vi "Mecanum_drive_edit.vi"(5 "practice bot":bool=TRUE, 6 "Rotation":dbl, 7 "Gyro Angle":dbl, 8 "error in (no error)":errorcluster, 9 "Y":dbl, 10 "X":dbl, 11 "RobotDriveDevRef":T1={"DevStatus"={"status"=FALSE, "code"=0, "source"=""}, "Motors[]"=[], "Square Inputs"=FALSE, "Max Output"=1.0}) -> (0 "error out":errorcluster, 2 "Motor Values":dbl[](array[numeric]), 3 "RobotDriveDevRef":T1={"DevStatus"={"status"=FALSE, "code"=0, "source"=""}, "Motors[]"=[], "Square Inputs"=FALSE, "Max Output"=1.0})   [LabVIEW 2014]
doc: "Configures the motors for holonomic driving. Holonomic driving allows you to move the robot in any direction without first rotating or maneuvering the robot.\n\nThis VI requires the robot to have either four omni-directional wheels and four motors mounted at 45 degree angles in the four corners of a square frame or to have four mecanum wheels driven by four motors.\n\nThe control input is intended to be connected directly to the X, Y, and Z axes of a joystick. The Y axis is inverted for you.\n\nThis software is licensed. Open the labview\\readme\\WPI Robotics Library Open Source License.txt file for more information."
uses:
  <vilib>/Rock Robotics/WPI/RobotDrive/WPI_RobotDriveDevRef.ctl
  <vilib>/Rock Robotics/WPI/MotorControl/WPI_MotorControlDeviceRef.ctl
  <vilib>/Rock Robotics/WPI/MotorControl/WPI_MotorControlType.ctl
  <vilib>/Rock Robotics/SystemInterfaces/Typedef/FPGA_TypedefDigitalModule.ctl
  <vilib>/Rock Robotics/SystemInterfaces/DIO/FPGA_DIOPWMChannel.ctl
  <vilib>/Rock Robotics/WPI/PWM/WPI_PWMDeadband.ctl
  <vilib>/Rock Robotics/WPI/CAN/Jaguar/SubVIs/WPI_CANJaguar_ControlMode.ctl
  <vilib>/Rock Robotics/WPI/CAN/TalonSRX/WPI_CANTalonSRX_APIControlMode.ctl
  <vilib>/Rock Robotics/WPI/PWM/WPI_PWMTransform_ConPane.ctl
  <vilib>/Rock Robotics/SystemInterfaces/NetworkCommunication/NetComm_UsageReport_ResourceType.ctl
  <vilib>/Rock Robotics/WPI/RobotDrive/WPI_RobotDriveMotorSelectorEnum.ctl
  <vilib>/Rock Robotics/WPI/Joystick/WPI_JoystickGetSetRefNum.vi
  <vilib>/Rock Robotics/WPI/RobotDrive/WPI_RobotDriveSafetyCheck.vi
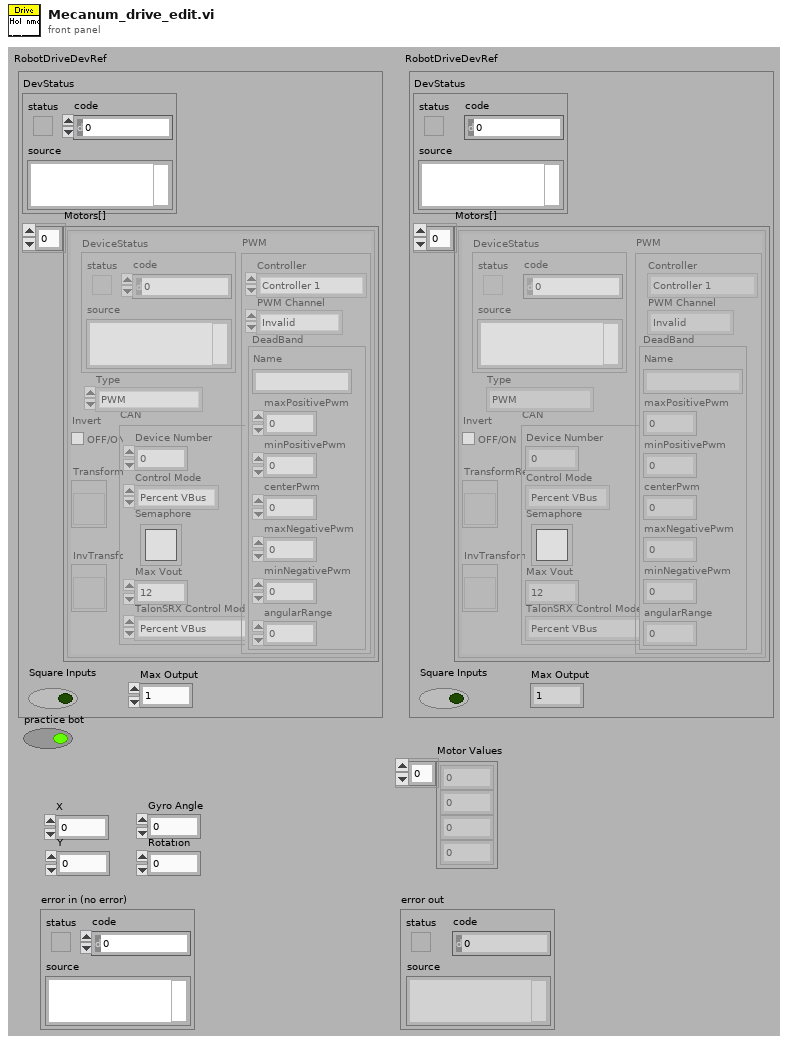
[diagram p1: front panel]
types:
  T1 = typedef "WPI_RobotDriveDevRef.ctl" = cluster{"DevStatus":errorcluster, "Motors[]":T2[], "Square Inputs":bool, "Max Output":dbl}
  T2 = typedef "WPI_MotorControlDeviceRef.ctl" = cluster{"DeviceStatus":errorcluster, "Type":T3, "PWM":cluster{"Controller":T4, "PWM Channel":T5, "DeadBand":T6}, "CAN":cluster{"Device Number":u8, "Control Mode":T7, "Semaphore":T8, "Max Vout":dbl, "TalonSRX Control Mode":T9}, "Invert":bool, "TransformRef":T10, "InvTransformRef":T10}
  T3 = typedef "WPI_MotorControlType.ctl" = enum16{"PWM", "CAN", "CANTalonSRX"}
  T4 = typedef "FPGA_TypedefDigitalModule.ctl" = enum16{"Controller 1"}
  T5 = typedef "FPGA_DIOPWMChannel.ctl" = enum8{"PWM 0", "PWM 1", "PWM 2", "PWM 3", "PWM 4", "PWM 5", "PWM 6", "PWM 7", "PWM 8", "PWM 9", "PWM MXP 0", "PWM MXP 1", "PWM MXP 2", "PWM MXP 3", "PWM MXP 4", "PWM MXP 5", "PWM MXP 6", "PWM MXP 7", "PWM MXP 8", "PWM MXP 9", "Invalid"}
  T6 = typedef "WPI_PWMDeadband.ctl" = cluster{"Name":string, "maxPositivePwm":i32, "minPositivePwm":i32, "centerPwm":i32, "maxNegativePwm":i32, "minNegativePwm":i32, "angularRange":u16}
  T7 = typedef "WPI_CANJaguar_ControlMode.ctl" = enum8{"Percent VBus", "Current", "Speed", "Position", "Voltage"}
  T8 = typedef "Semaphore RefNum" = refnum<k1>
  T9 = typedef "WPI_CANTalonSRX_APIControlMode.ctl" = enum8{"Percent VBus", "Speed", "Position", "Slave", "Unchanged / Invalid"}
  T10 = typedef "WPI_PWMTransform_ConPane.ctl" = refnum<vi>
  T11 = typedef "NetComm_UsageReport_ResourceType.ctl" = enum8{"Controller", "Module", "Language", "CANPlugin", "Accelerometer", "ADXL345", "AnalogChannel", "AnalogTrigger", "AnalogTriggerOutput", "CANJaguar", "Compressor", "Counter", "Dashboard", "DigitalInput", "DigitalOutput", "DriverStationCIO", "DriverStationEIO", "DriverStationLCD", "Encoder", "GearTooth", "Gyro", "I2C", "Framework", "Jaguar", "Joystick", "Kinect", "KinectStick", "PIDController", "Preferences", "PWM", "Relay", "RobotDrive", "SerialPort", "Servo", "Solenoid", "SPI", "Task", "Ultrasonic", "Victor", "Button", "Command", "AxisCamera", "PCVideoServer", "SmartDashboard", "Talon", "HiTechnicColorSensor", "HiTechnicAccel", "HiTechnicCompass", "SRF08", "AnalogOutput", "Victor SP", "Talon SRX", "CAN Talon SRX"}
  T12 = typedef "WPI_RobotDriveMotorSelectorEnum.ctl" = enum16{"Rear Left Motor", "Rear Right Motor", "Front Left Motor", "Front Right Motor"}
  T13 = typedef "WPI_JoystickDevRef.ctl" = cluster{"Device":T14}
  T14 = typedef "WPI_JoystickDeviceEnum.ctl" = enum16{"USB 0", "USB 1", "USB 2", "USB 3", "USB 4", "USB 5"}
  T15 = cluster{"Axes[0]":dbl, "Axes[1]":dbl, "Axes[2]":dbl, "Axes[3]":dbl, "Axes[4]":dbl, "Axes[5]":dbl, "Axes[6]":dbl, "Axes[7]":dbl, "Axes[8]":dbl}
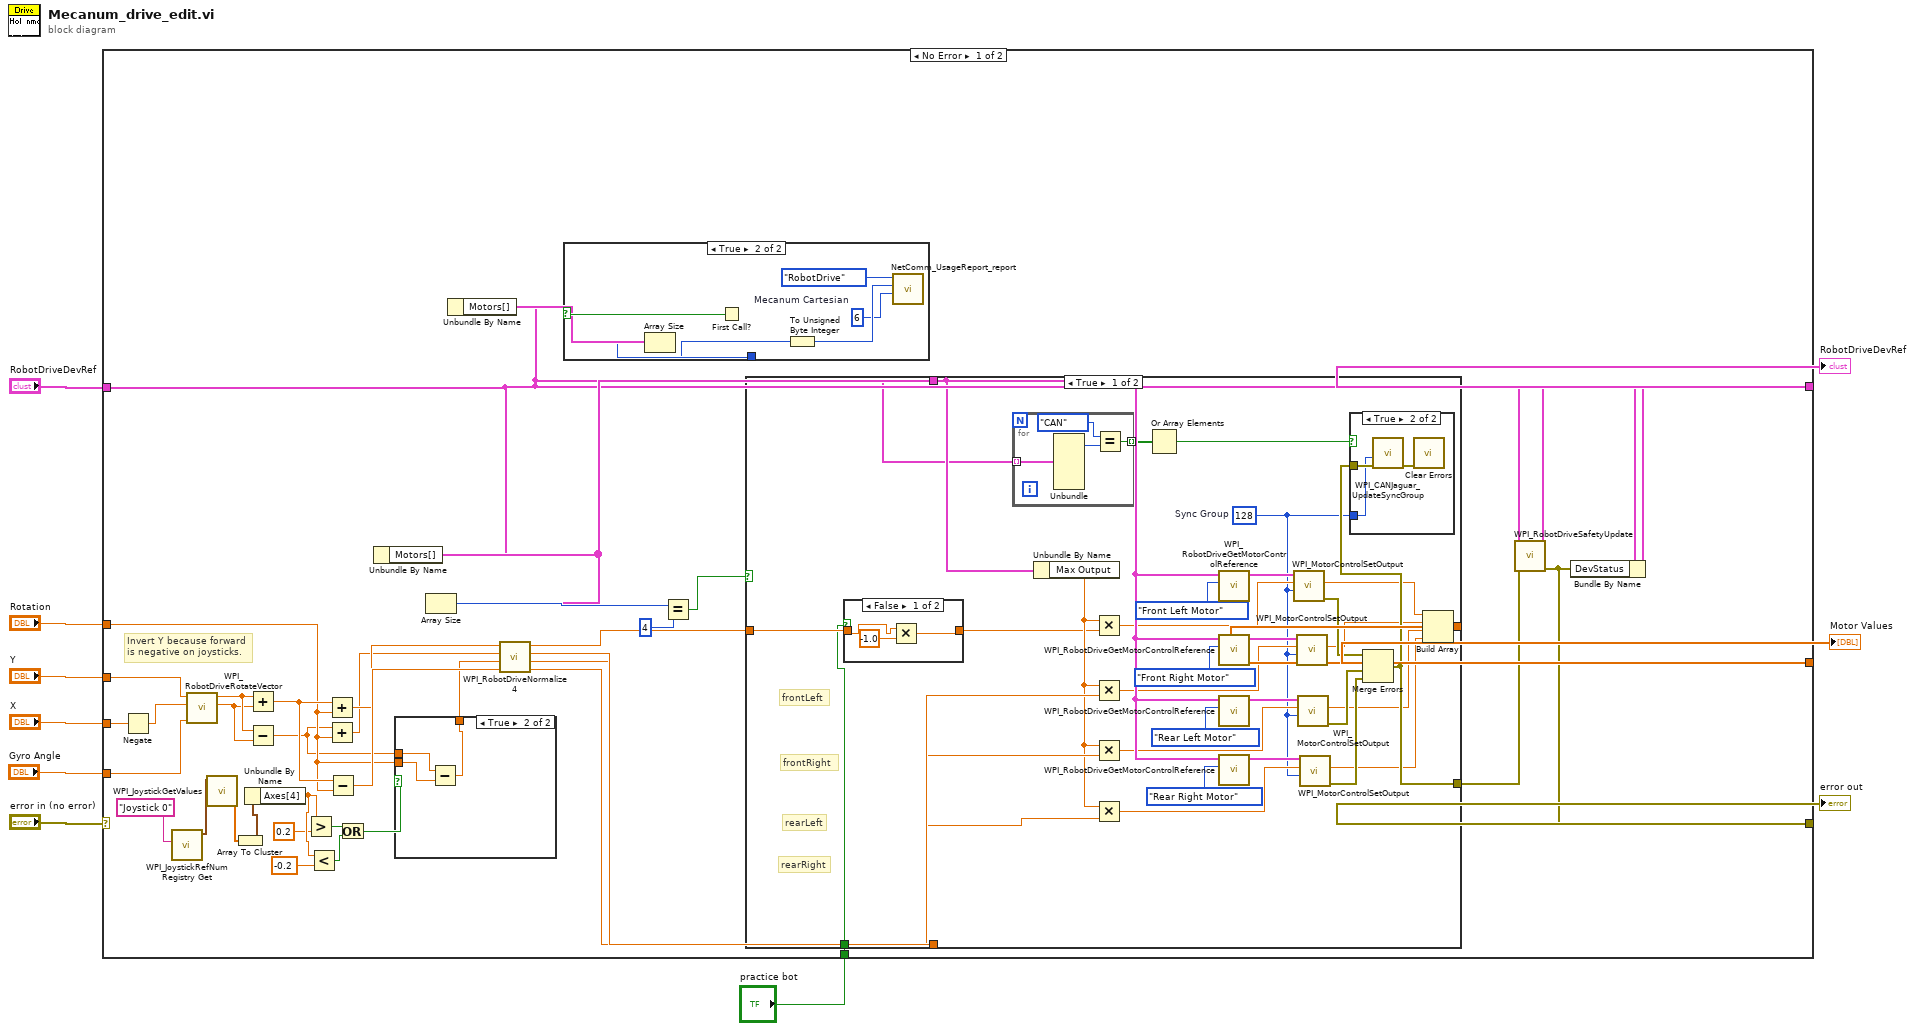
[diagram p0: block diagram]
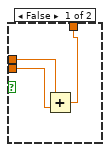
[diagram p2: hidden frame]
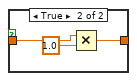
[diagram p4: hidden frame]
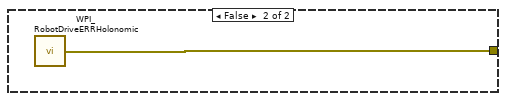
[diagram p6: hidden frame]
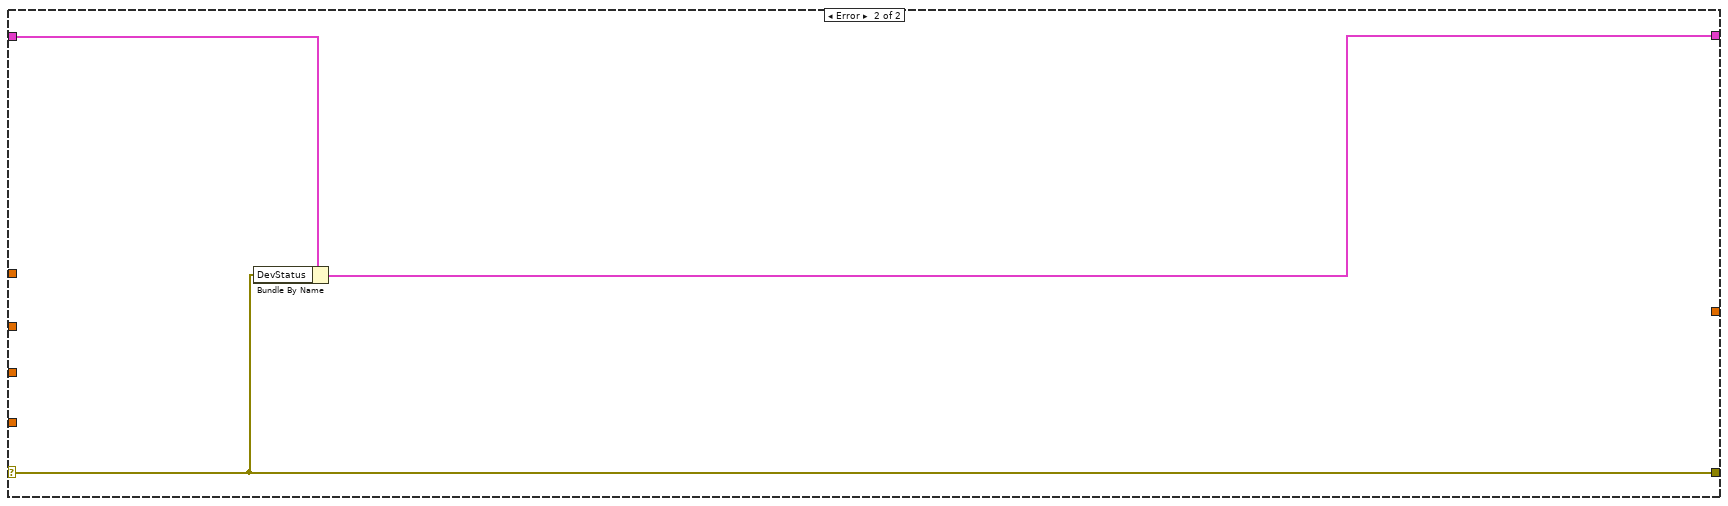
[diagram p7: hidden frame]
diagram:
  n1 = case shown="No Error" "error in (no error)" {
    selector: "error in (no error)" -> [_ w110]
    tunnel: "Y" -> [w14 _]
    tunnel: "X" -> [w12 _]
    tunnel: "RobotDriveDevRef" -> [w32 w112]
    tunnel: [w48 w111] -> w6
    tunnel: [w37 w110] -> w5
    tunnel: "Rotation" -> [w16 _]
    tunnel: "Gyro Angle" -> [w27 _]
    tunnel: [w31 _] -> w2
    tunnel: "practice bot" -> [w11 _]
    frame No Error {
      # "Invert Y because forward is negative on joysticks."
      n2 = Negate(x=w12) -> (-x=w13:dbl)
      n3 = call <vilib>:"WPI_JoystickRefNum Registry Get.vi"("refnum name"="Joystick 0") -> ("JoystickDevRef"=w29:T13)  [unwired: 9 in, 1 out]
      n4 = call <vilib>:"WPI_RobotDriveRotateVector.vi"("Angle"=w27, "X"=w13, "Y"=w14) -> ("X'"=w46:dbl, "Y'"=w47:dbl)  [unwired: 7 out]
      n5 = call <vilib>:"WPI_JoystickGetValues.vi"("JoystickDevRef"=w29) -> ("Axes"=w24:dbl[])  [unwired: 6 in, 4 out]
      n6 = Array To Cluster(array=w24) -> (cluster=w23:T15)
      n7 = Unbundle By Name(w23) -> ("Axes[4]"=w22:dbl)
      n8 = Add(x=w47, y=w46) -> (x+y=w19:dbl)
      n9 = Subtract(x=w47, y=w46) -> (x-y=w15:dbl)
      n10 = Greater?(x=w22, y=0.2) -> (0:w26:bool)
      n11 = Less?(x=w22, y=-0.2) -> (x < y?=w25:bool)
      n12 = Add(x=w19, y=w16) -> (x+y=w44:dbl)
      n13 = Add(x=w15, y=w16) -> (x+y=w30:dbl)
      n14 = Subtract(x=w19, y=w16) -> (x-y=w45:dbl)
      n15 = Or(x=w26, y=w25) -> (x .or. y?=w18:bool)
      n16 = Unbundle By Name(w32) -> ("Motors[]"=w36:T2[])
      n17 = case shown="True" w18 {
        tunnel: [w54 w55] -> w17
        tunnel: w16 -> [w53 w56]
        tunnel: w15 -> [w52 w57]
        frame False {
          n18 = Add(x=w52, y=w53) -> (x+y=w54:dbl)
        }
        frame True {
          n19 = Subtract(x=w57, y=w56) -> (x-y=w55:dbl)
        }
      }
      n20 = Array Size(array=w36) -> (size(s)=w51:i32)
      n21 = Unbundle By Name(w32) -> ("Motors[]"=w34:T2[])
      n22 = call <vilib>:"WPI_RobotDriveNormalize 4.vi"("D"=w45, "C"=w17, "B"=w30, "A"=w44) -> ("D'"=w41:dbl, "C'"=w40:dbl, "B'"=w42:dbl, "A'"=w43:dbl)
      n23 = Array Size(array=w34) -> (size(s)=w33:i32)
      n24 = Equal?(x=w51, y=4) -> (x = y?=w49:bool)
      n25 = First Call?() -> (First Call?: T/F=w35:bool)
      n26 = case shown="True" w35 {
        tunnel: w33 -> [_ w60]
        frame False {
        }
        frame True {
          w58 = u8 6  # Mecanum Cartesian
          n27 = To Unsigned Byte Integer(number=w60) -> (unsigned 8bit integer=w59:u8)
          n28 = call <vilib>:"NetComm_UsageReport_report.vi"("Context"=w58, "Instance Number"=w59, "Resource Type"=NetComm_UsageReport_ResourceType."RobotDrive") -> ()  [unwired: 9 in]
        }
      }
      n29 = case shown="True" w49 {
        tunnel: w43 -> [w65 _]
        tunnel: w42 -> [w95 _]
        tunnel: w32 -> [w85 _]
        tunnel: [w72 w109] -> w39
        tunnel: w40 -> [w90 _]
        tunnel: w41 -> [w63 _]
        tunnel: w36 -> [w73 _]
        tunnel: [w69 _] -> w31
        tunnel: w11 -> [w62 _]
        frame True {
          w71 = u8 128  # Sync Group
          # "rearLeft"
          # "frontRight"
          # "frontLeft"
          # "rearRight"
          n30 = case shown="False" w62 {
            tunnel: w65 -> [w96 w101]
            tunnel: [w97 w100] -> w64
            frame False {
              n31 = Multiply(x=w96, y=-1.0) -> (x*y=w97:dbl)
            }
            frame True {
              n32 = Multiply(x=w101, y=1.0) -> (x*y=w100:dbl)
            }
          }
          n33 = for {
            tunnel: w73 -> [w105] mode=indexing
            tunnel: [w102] -> w74 mode=indexing
            n34 = Unbundle(w105) -> ("Type"=w104:T3)  [unwired: 6 out]
            n35 = Equal?(x=enum16{"PWM", "CAN"}."CAN" ("Type"), y=w104) -> (x = y?=w102:bool)
          }
          n36 = Unbundle By Name(w85) -> ("Max Output"=w80:dbl)
          n37 = Multiply(x=w80, y=w64) -> (x*y=w84:dbl)
          n38 = Multiply(x=w80, y=w95) -> (x*y=w83:dbl)
          n39 = Multiply(x=w80, y=w90) -> (x*y=w82:dbl)
          n40 = Multiply(x=w80, y=w63) -> (x*y=w81:dbl)
          n41 = Or Array Elements(Boolean array=w74) -> (logical OR=w75:bool)
          n42 = call <vilib>:"WPI_RobotDriveGetMotorControlReference.vi"("MotorIndex"=WPI_RobotDriveMotorSelectorEnum."Front Left Motor", "RobotDriveDevRef"=w85) -> ("MotorControlDeviceRef"=w94:T2)  [unwired: 9 out]
          n43 = call <vilib>:"WPI_RobotDriveGetMotorControlReference.vi"("MotorIndex"=WPI_RobotDriveMotorSelectorEnum."Front Right Motor", "RobotDriveDevRef"=w85) -> ("MotorControlDeviceRef"=w92:T2)  [unwired: 9 out]
          n44 = call <vilib>:"WPI_RobotDriveGetMotorControlReference.vi"("MotorIndex"=WPI_RobotDriveMotorSelectorEnum."Rear Left Motor", "RobotDriveDevRef"=w85) -> ("MotorControlDeviceRef"=w93:T2)  [unwired: 9 out]
          n45 = call <vilib>:"WPI_RobotDriveGetMotorControlReference.vi"("MotorIndex"=WPI_RobotDriveMotorSelectorEnum."Rear Right Motor", "RobotDriveDevRef"=w85) -> ("MotorControlDeviceRef"=w91:T2)  [unwired: 9 out]
          n46 = call <vilib>:"WPI_MotorControlSetOutput.vi"("Sync Group / Parameter Slot"=w71, "Output"=w84, "MotorControlDevRef"=w94) -> ("error out"=w76:errorcluster, "Motor Output"=w70:dbl)  [unwired: 2 in, 5 out]
          n47 = call <vilib>:"WPI_MotorControlSetOutput.vi"("Sync Group / Parameter Slot"=w71, "Output"=w83, "MotorControlDevRef"=w92) -> ("error out"=w77:errorcluster, "Motor Output"=w68:dbl)  [unwired: 2 in, 5 out]
          n48 = call <vilib>:"WPI_MotorControlSetOutput.vi"("Sync Group / Parameter Slot"=w71, "Output"=w82, "MotorControlDevRef"=w93) -> ("error out"=w78:errorcluster, "Motor Output"=w67:dbl)  [unwired: 2 in, 5 out]
          n49 = call <vilib>:"WPI_MotorControlSetOutput.vi"("Sync Group / Parameter Slot"=w71, "Output"=w81, "MotorControlDevRef"=w91) -> ("error out"=w79:errorcluster, "Motor Output"=w66:dbl)  [unwired: 2 in, 5 out]
          n50 = Merge Errors(w76, w77, w78, w79) -> (w72:errorcluster)
          n51 = case shown="True" w75 {
            tunnel: w72 -> [_ w107]
            tunnel: w71 -> [_ w106]
            frame False {
            }
            frame True {
              n52 = call <vilib>:"WPI_CANJaguar_UpdateSyncGroup.vi"("error in (no error)"=w107, "Sync Group"=w106) -> ("error out"=w108:errorcluster)  [unwired: 9 out]
              n53 = call <vilib>:"Clear Errors.vi"("error in (no error)"=w108) -> ()  [unwired: 1 in, 6 out]
            }
          }
          n54 = Build Array(w70, w68, w67, w66) -> (w69:dbl[])
        }
        frame False {
          n55 = call <vilib>:"WPI_RobotDriveERRHolonomic.vi"() -> ("error out"=w109:errorcluster)
        }
      }
      n56 = call <vilib>:"WPI_RobotDriveSafetyUpdate.vi"("error in (no error)"=w39, "RobotDriveDevRef"=w32) -> ("error out"=w37:errorcluster, "RobotDriveDevRef"=w38:T1)  [unwired: 8 out]
      n57 = Bundle By Name(cluster=w38, "DevStatus"=w37) -> (w48:T1)
    }
    frame Error {
      n58 = Bundle By Name(cluster=w112, "DevStatus"=w110) -> (w111:T1)
    }
  }
  "error out" <- w5
  "RobotDriveDevRef" <- w6
  "Motor Values" <- w2
